vi "-8213 Invalid Virtual Instrument Identifier--error.vi"(8 "error in":errorcluster, 11 "Virtual Instrument Identifier":string) -> (0 "error out":errorcluster)   [LabVIEW 2024, in "Instrument Manager.lvclass"]
uses:
  Instrument Manager.lvclass
  Instrument Manager.lvclass/Instrument Manager.ctl
  Common-LabVIEW-Helpers/Source/Error Helpers.lvlib
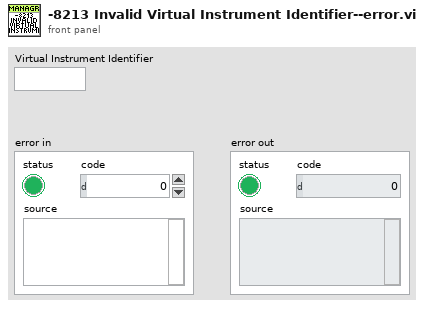
[diagram p1: front panel]
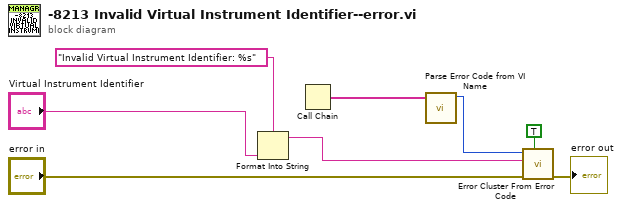
[diagram p0: block diagram]
diagram:
  n1 = Format Into String(format string="Invalid Virtual Instrument Identifier: %s", "Virtual Instrument Identifier") -> (resulting string=w7:string)  [unwired: 2 in, 1 out]
  n2 = Call Chain() -> (call chain=w2:string[])
  n3 = call "Parse Error Code from VI Name.vi"("Call Chain"=w2) -> ("Error Code"=w1:i32)  [unwired: 10 in]
  n4 = call <vilib>:"Error Cluster From Error Code.vi"("show call chain? (False)"=TRUE, "error in (no error)"="error in", "error message (\"\")"=w7, "error code (0)"=w1) -> ("error out"=→"error out":errorcluster)  [unwired: 5 in]
